vi "Auto Mast.vi"   [LabVIEW 2018]
uses:
  <vilib>/Rock Robotics/Network Tables/NT Read Number.vi
  <vilib>/Rock Robotics/Network Tables/NT Read Boolean.vi
  <vilib>/Rock Robotics/Network Tables/NT Write Boolean.vi
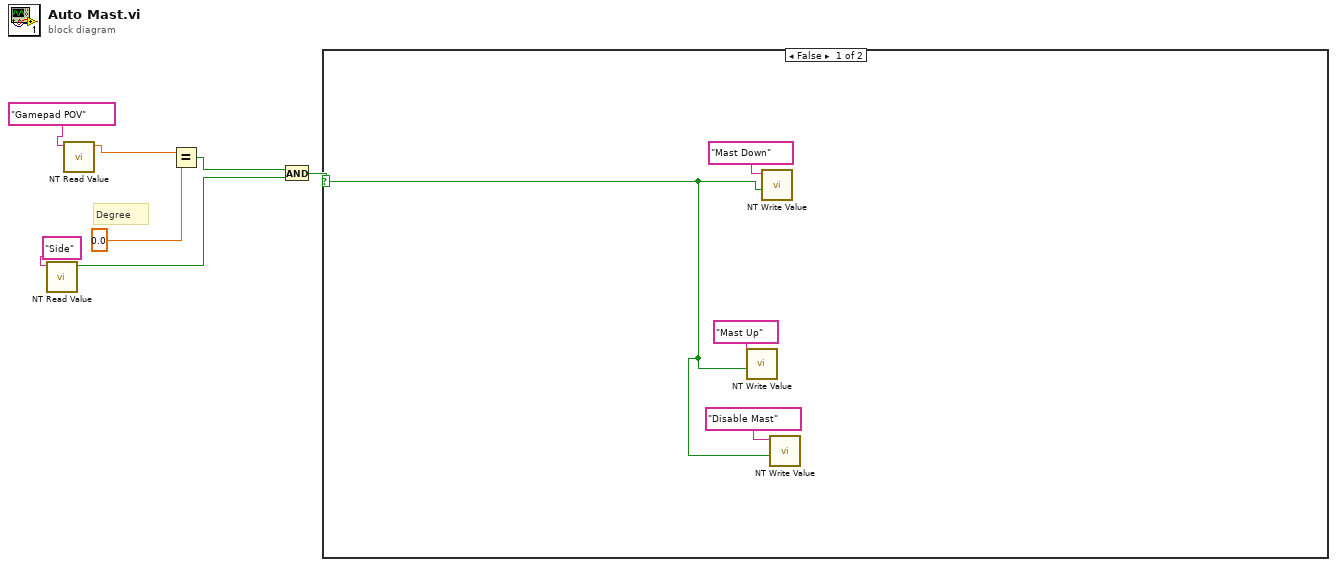
[diagram p0: block diagram]
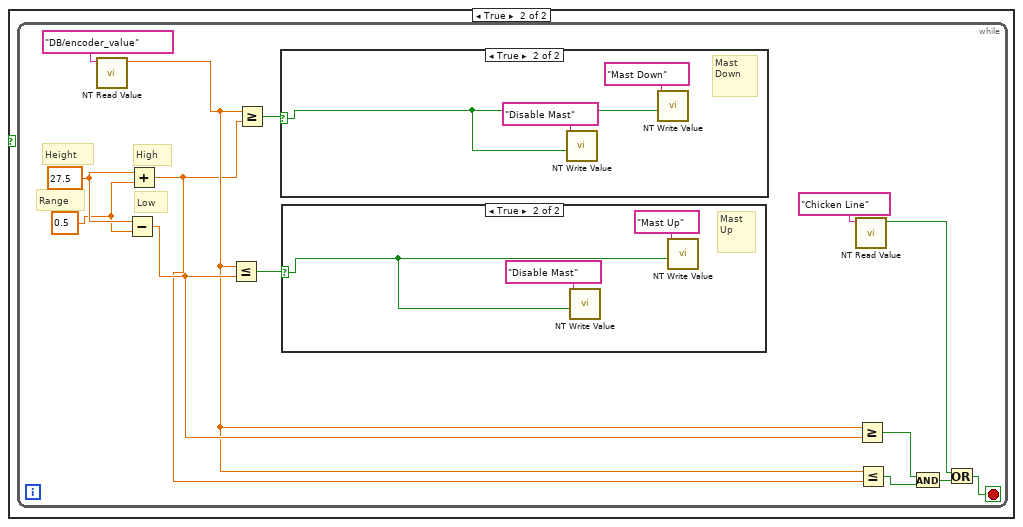
[diagram p2: hidden frame]
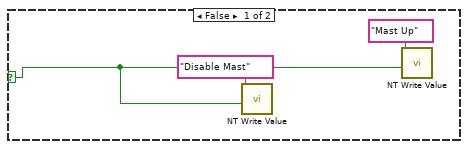
[diagram p3: hidden frame]
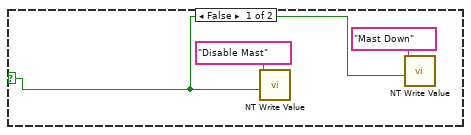
[diagram p4: hidden frame]
diagram:
  # "Degree"
  n1 = call-poly <vilib>:"NT Read Value.vi"("Name"="Side") -> ("Boolean"=w3:bool)  [unwired: 9 in, 1 out]
  n2 = call-poly <vilib>:"NT Read Value.vi"("Name"="Gamepad POV") -> ("Numeric"=w6:dbl)  [unwired: 9 in, 1 out]
  n3 = Equal?(x=w6, y=0.0) -> (x = y?=w2:bool)
  n4 = And(x=w2, y=w3) -> (x .and. y?=w1:bool)
  n5 = case shown="False" w1 {
    selector: w1 -> [w8 _]
    frame False {
      n6 = call-poly <vilib>:"NT Write Value.vi"("Boolean"=w8, "Name"="Mast Up") -> ()  [unwired: 9 in, 1 out]
      n7 = call-poly <vilib>:"NT Write Value.vi"("Boolean"=w8, "Name"="Mast Down") -> ()  [unwired: 9 in, 1 out]
      n8 = call-poly <vilib>:"NT Write Value.vi"("Boolean"=w8, "Name"="Disable Mast") -> ()  [unwired: 9 in, 1 out]
    }
    frame True {
      n9 = while {
        stop <- w19 stop-if-true
        w23 = 0.5
        w24 = 27.5
        # "Low"
        # "High"
        # "Range"
        # "Height"
        n10 = call-poly <vilib>:"NT Read Value.vi"("Name"="DB/encoder_value") -> ("Numeric"=w13:dbl)  [unwired: 9 in, 1 out]
        n11 = Subtract(x=w24, y=w23) -> (x-y=w15:dbl)
        n12 = Add(x=w24, y=w23) -> (x+y=w12:dbl)
        n13 = Less Or Equal?(x=w13, y=w15) -> (x <= y?=w22:bool)
        n14 = Greater Or Equal?(x=w13, y=w12) -> (x >= y?=w21:bool)
        n15 = case shown="True" w21 {
          selector: w21 -> [w32 w35]
          frame False {
            n16 = call-poly <vilib>:"NT Write Value.vi"("Boolean"=w32, "Name"="Disable Mast") -> ()  [unwired: 9 in, 1 out]
            n17 = call-poly <vilib>:"NT Write Value.vi"("Boolean"=w32, "Name"="Mast Down") -> ()  [unwired: 9 in, 1 out]
          }
          frame True {
            # "Mast\nDown"
            n18 = call-poly <vilib>:"NT Write Value.vi"("Boolean"=w35, "Name"="Disable Mast") -> ()  [unwired: 9 in, 1 out]
            n19 = call-poly <vilib>:"NT Write Value.vi"("Boolean"=w35, "Name"="Mast Down") -> ()  [unwired: 9 in, 1 out]
          }
        }
        n20 = case shown="True" w22 {
          selector: w22 -> [w26 w29]
          frame False {
            n21 = call-poly <vilib>:"NT Write Value.vi"("Boolean"=w26, "Name"="Disable Mast") -> ()  [unwired: 9 in, 1 out]
            n22 = call-poly <vilib>:"NT Write Value.vi"("Boolean"=w26, "Name"="Mast Up") -> ()  [unwired: 9 in, 1 out]
          }
          frame True {
            # "Mast\nUp"
            n23 = call-poly <vilib>:"NT Write Value.vi"("Boolean"=w29, "Name"="Disable Mast") -> ()  [unwired: 9 in, 1 out]
            n24 = call-poly <vilib>:"NT Write Value.vi"("Boolean"=w29, "Name"="Mast Up") -> ()  [unwired: 9 in, 1 out]
          }
        }
        n25 = call-poly <vilib>:"NT Read Value.vi"("Name"="Chicken Line") -> ("Boolean"=w18:bool)  [unwired: 9 in, 1 out]
        n26 = Greater Or Equal?(x=w13, y=w15) -> (x >= y?=w16:bool)
        n27 = Less Or Equal?(x=w13, y=w12) -> (x <= y?=w14:bool)
        n28 = And(x=w16, y=w14) -> (x .and. y?=w17:bool)
        n29 = Or(x=w18, y=w17) -> (x .or. y?=w19:bool)
      }
    }
  }
